vi "PXDAC4800_GetErrorMessXD48.vi"(0 "Handle":u32, 5 "Flags":i32=1, 7 "Error":i32) -> (4 "ErrMess":string)   [LabVIEW 2016]
uses:
  PXDAC4800.dll
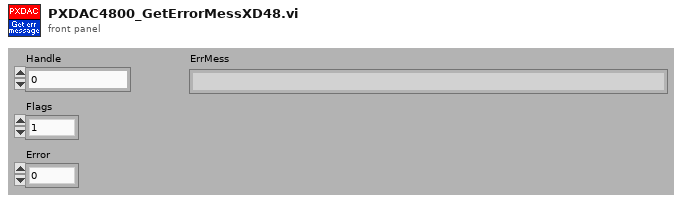
[diagram p1: front panel]
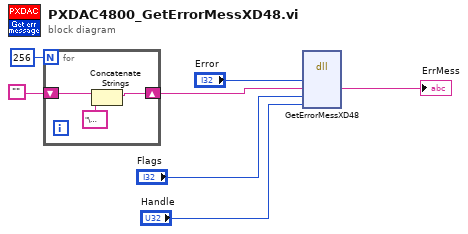
[diagram p0: block diagram]
diagram:
  n1 = for {
    N: 256 -> [_]
    shift-right: [w9] -> w2
    shift-left: "" -> [w10]
    n2 = Concatenate Strings(w10, "\u0000") -> (w9:string)
  }
  n3 = dll-call lib="PXDAC4800.dll" fn="GetErrorMessXD48"("Error"="Error", "ErrMess"=w2, "Flags"="Flags", "Handle"="Handle") -> ("ErrMess"=→"ErrMess":string)  [unwired: 7 in, 2 out]
